vi "E7_20_readstring.vi"(1 "read buffer":string, 5 "Error In":errorcluster) -> (6 "Offset":dbl, 8 "Level":dbl, 9 "Error Out":errorcluster, 10 "Frequency":dbl, 11 "SecParam":dbl, 12 "FLAGS":dbl, 13 "ImParam":dbl, 14 "Mode":dbl, 15 "CS":dbl, 16 "OnChange":dbl, 17 "Limit":dbl, 18 "ImParam_Value":dbl, 19 "SecParam_Value":dbl)   [LabVIEW 2018]
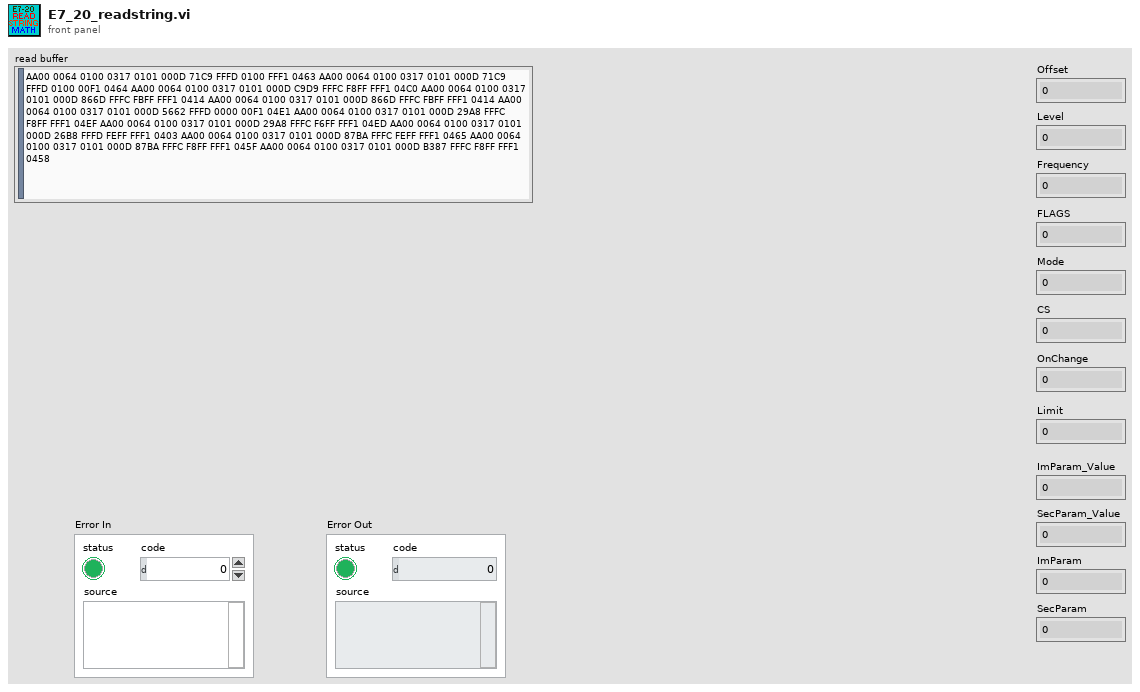
[diagram p1: front panel]
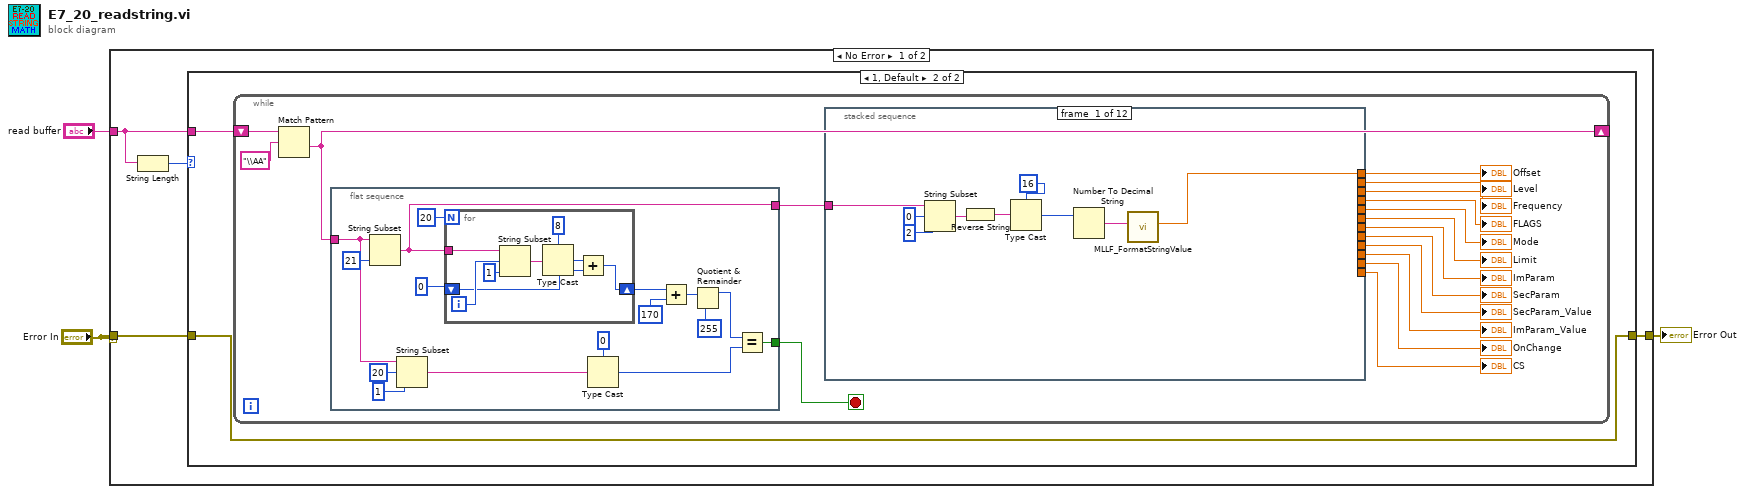
[diagram p0: block diagram]
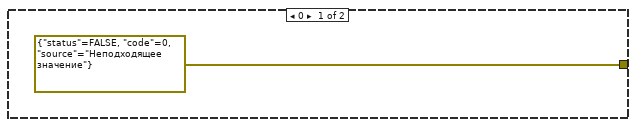
[diagram p2: hidden frame]
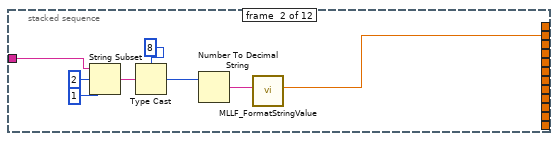
[diagram p3: hidden frame]
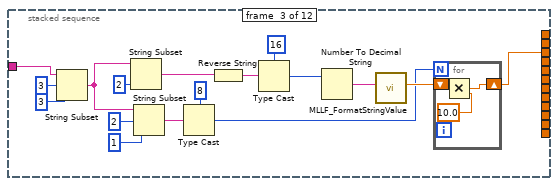
[diagram p4: hidden frame]
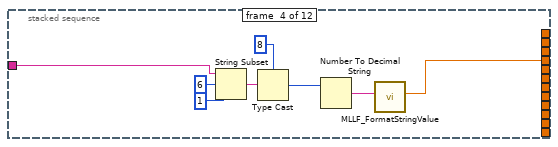
[diagram p5: hidden frame]
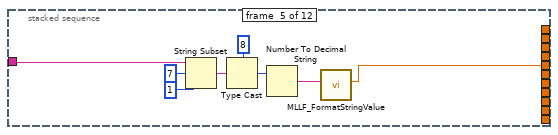
[diagram p6: hidden frame]
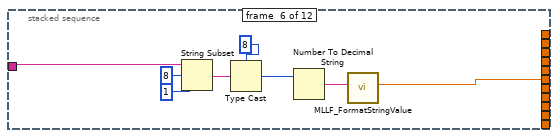
[diagram p7: hidden frame]
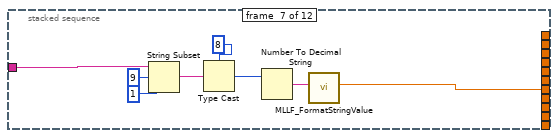
[diagram p8: hidden frame]
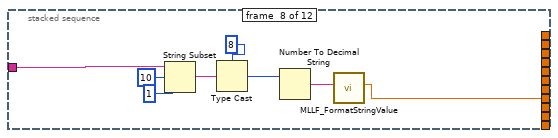
[diagram p9: hidden frame]
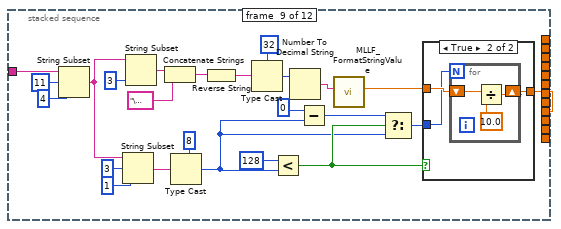
[diagram p10: hidden frame]
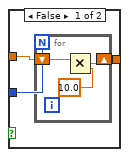
[diagram p11: hidden frame]
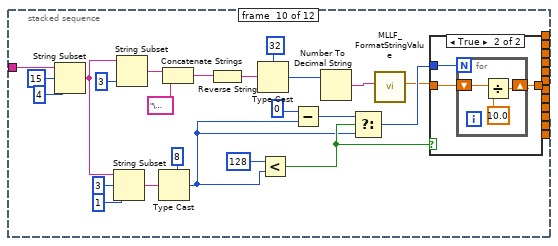
[diagram p12: hidden frame]
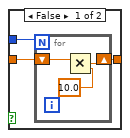
[diagram p13: hidden frame]
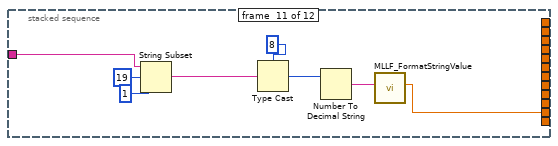
[diagram p14: hidden frame]
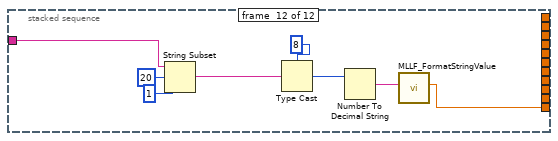
[diagram p15: hidden frame]
diagram:
  n1 = case shown="No Error" "Error In" {
    tunnel: "read buffer" -> [w7 _]
    tunnel: "Error In" -> [w4 w217]
    tunnel: [w5 w217] -> w2
    frame No Error {
      n2 = String Length(string=w7) -> (length=w6:i32)
      n3 = case shown="1, Default" w6 {
        tunnel: w7 -> [_ w10]
        tunnel: [errorcluster {"status"=FALSE, "code"=0, "source"="Неподходящее значение"} ("Error In") w9] -> w5
        tunnel: w4 -> [_ w9]
        frame 0 {
        }
        frame 1, Default {
          n4 = while {
            shift-right: [w25] -> _
            shift-left: w10 -> [w26]
            stop <- w24 stop-if-true
            n5 = Match Pattern(string=w26, regular expression="\\AA") -> (after substring=w25:string)  [unwired: 1 in, 3 out]
            n6 = flat-sequence {
              tunnel: w25 -> [w38]
              tunnel: [w31] -> w24
              tunnel: [w30] -> w23
              frame #0 {
                n7 = String Subset(string=w38, length (rest)=21 ("length (rest)")) -> (substring=w30:string)  [unwired: 1 in]
                n8 = String Subset(string=w38, offset (0)=20, length (rest)=1 ("length (rest)")) -> (substring=w39:string)
                n9 = for {
                  N: 20 ("length (rest)") -> [_]
                  tunnel: w30 -> [w45]
                  shift-right: [w46] -> w37
                  shift-left: u8 0 -> [w47]
                  i -> [w50]
                  n10 = String Subset(string=w45, offset (0)=w50, length (rest)=1 ("length (rest)")) -> (substring=w48:string)
                  n11 = Type Cast(type=u8 8, x=w48) -> (*(type *) &x=w44:u8)
                  n12 = Add(x=w44, y=w47) -> (x+y=w46:u8)
                }
                n13 = Type Cast(type=u8 0, x=w39) -> (*(type *) &x=w29:u8)
                n14 = Add(x=w37, y=u8 170 ("length (rest)")) -> (x+y=w36:u8)
                n15 = Quotient & Remainder(x=w36, y=u8 255 ("length (rest)")) -> (x-y*floor(x/y)=w28:u8)  [unwired: 1 out]
                n16 = Equal?(x=w28, y=w29) -> (x = y?=w31:bool)
              }
            }
            n17 = stacked-sequence {
              tunnel: w23 -> [w55 w63 w70 w90 w98 w106 w114 w122 w130 w166 w202 w210]
              tunnel: [_ _ _ _ _ _ _ _ w129 _ _ _] -> w22
              tunnel: [_ _ _ _ _ _ _ _ _ _ w201 _] -> w21
              tunnel: [_ _ _ _ _ _ _ _ _ _ _ w209] -> w20
              tunnel: [w52 _ _ _ _ _ _ _ _ _ _ _] -> w19
              tunnel: [_ w61 _ _ _ _ _ _ _ _ _ _] -> w18
              tunnel: [_ _ w69 _ _ _ _ _ _ _ _ _] -> w17
              tunnel: [_ _ _ w89 _ _ _ _ _ _ _ _] -> w16
              tunnel: [_ _ _ _ w97 _ _ _ _ _ _ _] -> w15
              tunnel: [_ _ _ _ _ _ w113 _ _ _ _ _] -> w14
              tunnel: [_ _ _ _ _ _ _ w121 _ _ _ _] -> w13
              tunnel: [_ _ _ _ _ _ _ _ _ w165 _ _] -> w12
              tunnel: [_ _ _ _ _ w105 _ _ _ _ _ _] -> w11
              frame #0 {
                n18 = String Subset(string=w55, offset (0)=0 ("length (rest)"), length (rest)=2 ("length (rest)")) -> (substring=w60:string)
                n19 = Reverse String(1:w60) -> (0:w58:string)
                n20 = Type Cast(type=u16 16, x=w58) -> (*(type *) &x=w53:u16)
                n21 = Number To Decimal String(number=w53) -> (decimal integer string=w59:string)  [unwired: 1 in]
                n22 = call "MLLF_FormatStringValue.vi"("String Value"=w59) -> ("number"=w52:dbl)  [unwired: 8 in, 2 out]
              }
              frame #1 {
                n23 = String Subset(string=w63, offset (0)=2 ("length (rest)"), length (rest)=1 ("length (rest)")) -> (substring=w68:string)
                n24 = Type Cast(type=u8 8, x=w68) -> (*(type *) &x=w67:u8)
                n25 = Number To Decimal String(number=w67) -> (decimal integer string=w66:string)  [unwired: 1 in]
                n26 = call "MLLF_FormatStringValue.vi"("String Value"=w66) -> ("number"=w61:dbl)  [unwired: 8 in, 2 out]
              }
              frame #2 {
                n27 = String Subset(string=w70, offset (0)=3 ("length (rest)"), length (rest)=3 ("length (rest)")) -> (substring=w83:string)
                n28 = String Subset(string=w83, length (rest)=2 ("length (rest)")) -> (substring=w85:string)  [unwired: 1 in]
                n29 = String Subset(string=w83, offset (0)=2, length (rest)=1 ("length (rest)")) -> (substring=w76:string)
                n30 = Type Cast(type=u8 8, x=w76) -> (*(type *) &x=w77:u8)
                n31 = Reverse String(1:w85) -> (0:w80:string)
                n32 = Type Cast(type=u16 16, x=w80) -> (*(type *) &x=w82:u16)
                n33 = Number To Decimal String(number=w82) -> (decimal integer string=w81:string)  [unwired: 1 in]
                n34 = call "MLLF_FormatStringValue.vi"("String Value"=w81) -> ("number"=w84:dbl)  [unwired: 8 in, 2 out]
                n35 = for {
                  N: w77 -> [_]
                  shift-right: [w88] -> w69
                  shift-left: w84 -> [w86]
                  n36 = Multiply(x=w86, y=10.0) -> (x*y=w88:dbl)
                }
              }
              frame #3 {
                n37 = String Subset(string=w90, offset (0)=6 ("length (rest)"), length (rest)=1 ("length (rest)")) -> (substring=w95:string)
                n38 = Type Cast(type=u8 8, x=w95) -> (*(type *) &x=w94:u8)
                n39 = Number To Decimal String(number=w94) -> (decimal integer string=w93:string)  [unwired: 1 in]
                n40 = call "MLLF_FormatStringValue.vi"("String Value"=w93) -> ("number"=w89:dbl)  [unwired: 8 in, 2 out]
              }
              frame #4 {
                n41 = String Subset(string=w98, offset (0)=7 ("length (rest)"), length (rest)=1 ("length (rest)")) -> (substring=w104:string)
                n42 = Type Cast(type=u8 8, x=w104) -> (*(type *) &x=w102:u8)
                n43 = Number To Decimal String(number=w102) -> (decimal integer string=w101:string)  [unwired: 1 in]
                n44 = call "MLLF_FormatStringValue.vi"("String Value"=w101) -> ("number"=w97:dbl)  [unwired: 8 in, 2 out]
              }
              frame #5 {
                n45 = String Subset(string=w106, offset (0)=8 ("length (rest)"), length (rest)=1 ("length (rest)")) -> (substring=w107:string)
                n46 = Type Cast(type=u8 8, x=w107) -> (*(type *) &x=w109:u8)
                n47 = Number To Decimal String(number=w109) -> (decimal integer string=w110:string)  [unwired: 1 in]
                n48 = call "MLLF_FormatStringValue.vi"("String Value"=w110) -> ("number"=w105:dbl)  [unwired: 8 in, 2 out]
              }
              frame #6 {
                n49 = String Subset(string=w114, offset (0)=9 ("length (rest)"), length (rest)=1 ("length (rest)")) -> (substring=w115:string)
                n50 = Type Cast(type=u8 8, x=w115) -> (*(type *) &x=w117:u8)
                n51 = Number To Decimal String(number=w117) -> (decimal integer string=w118:string)  [unwired: 1 in]
                n52 = call "MLLF_FormatStringValue.vi"("String Value"=w118) -> ("number"=w113:dbl)  [unwired: 8 in, 2 out]
              }
              frame #7 {
                n53 = String Subset(string=w122, offset (0)=10 ("length (rest)"), length (rest)=1 ("length (rest)")) -> (substring=w123:string)
                n54 = Type Cast(type=u8 8, x=w123) -> (*(type *) &x=w125:u8)
                n55 = Number To Decimal String(number=w125) -> (decimal integer string=w126:string)  [unwired: 1 in]
                n56 = call "MLLF_FormatStringValue.vi"("String Value"=w126) -> ("number"=w121:dbl)  [unwired: 8 in, 2 out]
              }
              frame #8 {
                n57 = String Subset(string=w130, offset (0)=11 ("length (rest)"), length (rest)=4 ("length (rest)")) -> (substring=w150:string)
                n58 = String Subset(string=w150, offset (0)=3, length (rest)=1 ("length (rest)")) -> (substring=w134:string)
                n59 = String Subset(string=w150, length (rest)=3 ("length (rest)")) -> (substring=w152:string)  [unwired: 1 in]
                n60 = Concatenate Strings(w152, "\u0000" ("string")) -> (w138:string)
                n61 = Type Cast(type=u8 8, x=w134) -> (*(type *) &x=w145:u8)
                n62 = Reverse String(1:w138) -> (0:w140:string)
                n63 = Type Cast(type=u32 32, x=w140) -> (*(type *) &x=w151:u32)
                n64 = Less?(x=u8 128, y=w145) -> (x < y?=w146:bool)
                n65 = Number To Decimal String(number=w151) -> (decimal integer string=w141:string)  [unwired: 1 in]
                n66 = Subtract(x=u8 0, y=w145) -> (x-y=w143:u8)
                n67 = call "MLLF_FormatStringValue.vi"("String Value"=w141) -> ("number"=w142:dbl)  [unwired: 8 in, 2 out]
                n68 = Select(t=w143, s=w146, f=w145) -> (s? t:f=w147:u8)
                n69 = case shown="True" w146 {
                  tunnel: w142 -> [w155 w161]
                  tunnel: [w154 w160] -> w129
                  tunnel: w147 -> [w153 w159]
                  frame False {
                    n70 = for {
                      N: w153 -> [_]
                      shift-right: [w158] -> w154
                      shift-left: w155 -> [w156]
                      n71 = Multiply(x=w156, y=10.0) -> (x*y=w158:dbl)
                    }
                  }
                  frame True {
                    n72 = for {
                      N: w159 -> [_]
                      shift-right: [w162] -> w160
                      shift-left: w161 -> [w164]
                      n73 = Divide(x=w164, y=10.0) -> (x/y=w162:dbl)
                    }
                  }
                }
              }
              frame #9 {
                n74 = String Subset(string=w166, offset (0)=15 ("length (rest)"), length (rest)=4 ("length (rest)")) -> (substring=w170:string)
                n75 = String Subset(string=w170, offset (0)=3, length (rest)=1 ("length (rest)")) -> (substring=w173:string)
                n76 = String Subset(string=w170, length (rest)=3 ("length (rest)")) -> (substring=w177:string)  [unwired: 1 in]
                n77 = Type Cast(type=u8 8, x=w173) -> (*(type *) &x=w186:u8)
                n78 = Concatenate Strings(w177, "\u0000" ("string")) -> (w178:string)
                n79 = Reverse String(1:w178) -> (0:w181:string)
                n80 = Type Cast(type=u32 32, x=w181) -> (*(type *) &x=w180:u32)
                n81 = Less?(x=u8 128, y=w186) -> (x < y?=w187:bool)
                n82 = Subtract(x=u8 0, y=w186) -> (x-y=w184:u8)
                n83 = Number To Decimal String(number=w180) -> (decimal integer string=w182:string)  [unwired: 1 in]
                n84 = Select(t=w184, s=w187, f=w186) -> (s? t:f=w188:u8)
                n85 = call "MLLF_FormatStringValue.vi"("String Value"=w182) -> ("number"=w183:dbl)  [unwired: 8 in, 2 out]
                n86 = case shown="True" w187 {
                  tunnel: w183 -> [w191 w197]
                  tunnel: [w190 w196] -> w165
                  tunnel: w188 -> [w189 w195]
                  frame False {
                    n87 = for {
                      N: w189 -> [_]
                      shift-right: [w194] -> w190
                      shift-left: w191 -> [w192]
                      n88 = Multiply(x=w192, y=10.0) -> (x*y=w194:dbl)
                    }
                  }
                  frame True {
                    n89 = for {
                      N: w195 -> [_]
                      shift-right: [w198] -> w196
                      shift-left: w197 -> [w200]
                      n90 = Divide(x=w200, y=10.0) -> (x/y=w198:dbl)
                    }
                  }
                }
              }
              frame #10 {
                n91 = String Subset(string=w202, offset (0)=19 ("length (rest)"), length (rest)=1 ("length (rest)")) -> (substring=w208:string)
                n92 = Type Cast(type=u8 8, x=w208) -> (*(type *) &x=w206:u8)
                n93 = Number To Decimal String(number=w206) -> (decimal integer string=w205:string)  [unwired: 1 in]
                n94 = call "MLLF_FormatStringValue.vi"("String Value"=w205) -> ("number"=w201:dbl)  [unwired: 8 in, 2 out]
              }
              frame #11 {
                n95 = String Subset(string=w210, offset (0)=20 ("length (rest)"), length (rest)=1 ("length (rest)")) -> (substring=w216:string)
                n96 = Type Cast(type=u8 8, x=w216) -> (*(type *) &x=w214:u8)
                n97 = Number To Decimal String(number=w214) -> (decimal integer string=w213:string)  [unwired: 1 in]
                n98 = call "MLLF_FormatStringValue.vi"("String Value"=w213) -> ("number"=w209:dbl)  [unwired: 8 in, 2 out]
              }
            }
            "SecParam_Value" <- w22
            "OnChange" <- w21
            "CS" <- w20
            "Offset" <- w19
            "Level" <- w18
            "Frequency" <- w17
            "FLAGS" <- w16
            "Mode" <- w15
            "ImParam" <- w14
            "SecParam" <- w13
            "ImParam_Value" <- w12
            "Limit" <- w11
          }
        }
      }
    }
    frame Error {
    }
  }
  "Error Out" <- w2
